vi "Actor Core.vi"(8 "error in":errorcluster, 11 "DisplayUI in":refnum<class "DisplayUI.lvclass">) -> (0 "error out":errorcluster, 3 "Actor out":refnum<class "Actor.lvclass">)   [LabVIEW 2013, in "DisplayUI.lvclass"]
doc: "(<B>Filename</B>: Actor Framework.lvlib:Actor.lvclass:Actor Core.vi)\n\nReceives messages to the actor, reacts to them, and initiates any error handling that may shut the actor down.\n\nDescendant classes may override this VI to append parallel tasks for the actor to complete while it handles messages. Overrides use the Call Parent Method node."
uses:
  DisplayUI.lvclass
  <vilib>/ActorFramework/Actor/Actor.lvclass
  <vilib>/ActorFramework/Actor/Actor.lvclass/Actor.ctl
  DisplayUI.lvclass/DisplayUI.ctl
  <vilib>/ActorFramework/Message Enqueuer/Message Enqueuer.lvclass/Message Enqueuer.ctl
  <vilib>/ActorFramework/Message Enqueuer/Enqueue.vi
  <vilib>/ActorFramework/Message Priority Queue/Priority Enqueue.vi
  Counter Messages/Increment Msg/Increment Msg.lvclass
  Counter Messages/DataToDisplay Msg/DataToDisplay Msg.lvclass
  Counter Messages/Decrement Msg/Decrement Msg.lvclass
panel:
  in  "DEC":bool
  in  "Exit":bool
  in  "INC":bool
  out "Count":i32
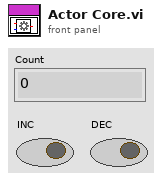
[diagram p1: front panel]
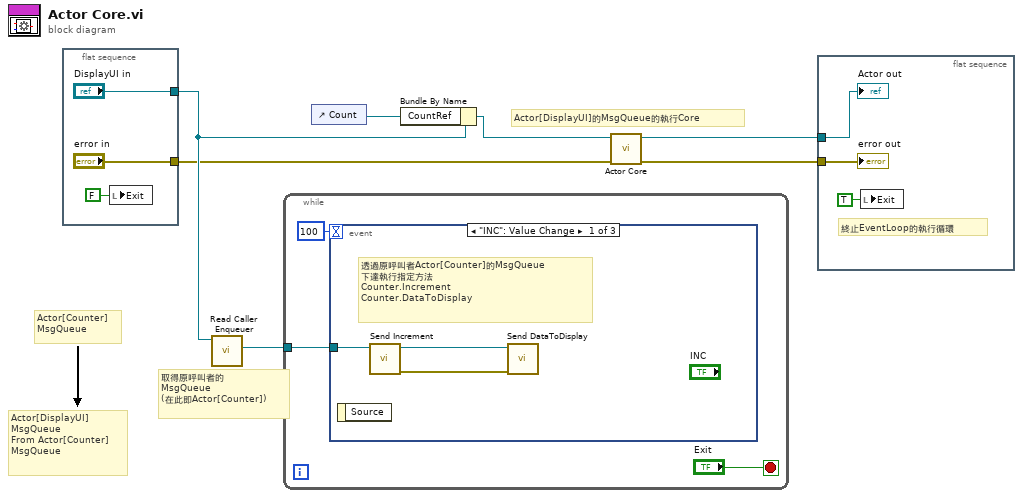
[diagram p0: block diagram]
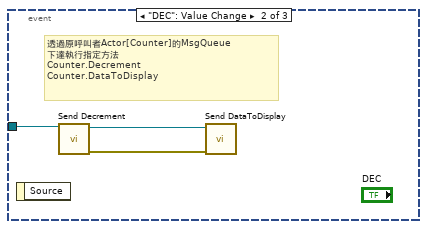
[diagram p2: hidden frame]
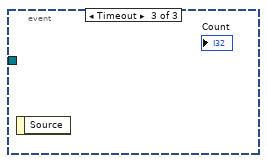
[diagram p3: hidden frame]
diagram:
  # "Actor[DisplayUI]的MsgQueue的執行Core"
  # "取得原呼叫者的\nMsgQueue\n(在此即Actor[Counter])"
  # "Actor[DisplayUI]\nMsgQueue\nFrom Actor[Counter]\nMsgQueue"
  # "Actor[Counter]\nMsgQueue"
  n1 = flat-sequence {
    tunnel: ["error in"] -> w1
    tunnel: ["DisplayUI in"] -> w4
    frame #0 {
      n2 = local write "Exit"(FALSE ("Exit")) -> ()
    }
  }
  n3 = call <vilib>:"Read Caller Enqueuer.vi"("Actor"=w4) -> ("Caller Enqueuer"=w5:refnum<class "Message Enqueuer.lvclass">)  [unwired: 10 in]
  n4 = while {
    tunnel: w5 -> [w13]
    stop <- "Exit" stop-if-true
    n5 = event shown="[0] \"INC\": Value Change" {
      selector: _ -> [_ _ _]
      dyn-events: _ -> [_ _ _]
      timeout: 100 -> [_ _ _]
      tunnel: w13 -> [w14 w17 _]
      event "INC": Value Change {
        # "透過原呼叫者Actor[Counter]的MsgQueue\n下達執行指定方法\nCounter.Increment\nCounter.DataToDisplay"
        n6 = event-data() -> ()  [unwired: 1 in, 1 out]
        n7 = call "Send Increment.vi"("Message Enqueuer"=w14) -> ("error out"=w15:errorcluster, "Message Enqueuer out"=w16:refnum<class "Message Enqueuer.lvclass">)  [unwired: 9 in]
        n8 = call "Send DataToDisplay.vi"("error in (no error)"=w15, "Message Enqueuer"=w16) -> ()  [unwired: 8 in, 2 out]
      }
      event "DEC": Value Change {
        # "透過原呼叫者Actor[Counter]的MsgQueue\n下達執行指定方法\nCounter.Decrement\nCounter.DataToDisplay"
        n9 = event-data() -> ()  [unwired: 1 in, 1 out]
        n10 = call "Send Decrement.vi"("Message Enqueuer"=w17) -> ("error out"=w19:errorcluster, "Message Enqueuer out"=w18:refnum<class "Message Enqueuer.lvclass">)  [unwired: 9 in]
        n11 = call "Send DataToDisplay.vi"("error in (no error)"=w19, "Message Enqueuer"=w18) -> ()  [unwired: 8 in, 2 out]
      }
      event Timeout {
        n12 = event-data() -> ()  [unwired: 1 in, 1 out]
      }
    }
  }
  n13 = control-ref of="Count"() -> (w3:refnum<vi>)
  n14 = Bundle By Name(cluster=w4, "CountRef"=w3) -> (w2:refnum<class "DisplayUI.lvclass">)
  n15 = call-parent "Actor Core.vi"("error in"=w1, "Actor in"=w2) -> ("error out"=w7:errorcluster, "Actor out"=w6:refnum<class "Actor.lvclass">)  [unwired: 8 in]
  n16 = flat-sequence {
    tunnel: w7 -> [w22]
    tunnel: w6 -> [w21]
    frame #0 {
      # "終止EventLoop的執行循環"
      n17 = local write "Exit"(TRUE ("Exit")) -> ()
      "error out" <- w22
      "Actor out" <- w21
    }
  }
